vi "bead-center-xy-correlation-simple-sum-v3.vi"(4 "Radial size":i32=64, 6 "Bead\nCoordinates":i32[](array[numeric])=[257, 440, 328, 479], 8 "error in (no error)":errorcluster caption="错误输入（无错误）", 9 "Scan Window Size":i32=40, 10 "Lines amount":i32=20, 11 "FullImage":T1) -> (0 "error out":errorcluster caption="错误输出", 1 "CoordinatesOut":i32[](array[numeric]), 2 "xy":dbl[](array[numeric]))   [LabVIEW 2013]
uses:
  <vilib>/vision/Image Controls.llb/IMAQ Image.ctl
panel:
  in  "传递变量":T2={"FullImage"=refnum, "Lines amount"=20, "Scan Window Size"=40, "Bead\nCoordinates"=[257, 440, 328, 479], "Radial size"=64, "center_X"=0.0, "center_Y"=0.0, "再次确认ROI"=FALSE}
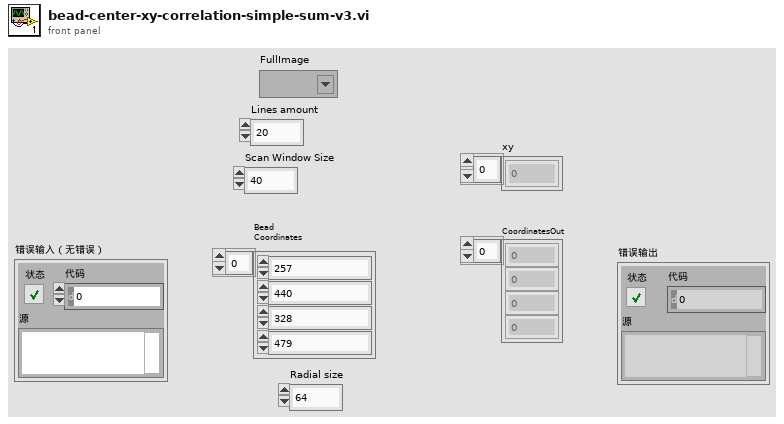
[diagram p1: front panel]
types:
  T1 = typedef "IMAQ Image.ctl" = refnum<image>
  T2 = cluster{"FullImage":T1, "Lines amount":i32, "Scan Window Size":i32, "Bead\nCoordinates":i32[], "Radial size":i32, "center_X":dbl, "center_Y":dbl, "再次确认ROI":bool}
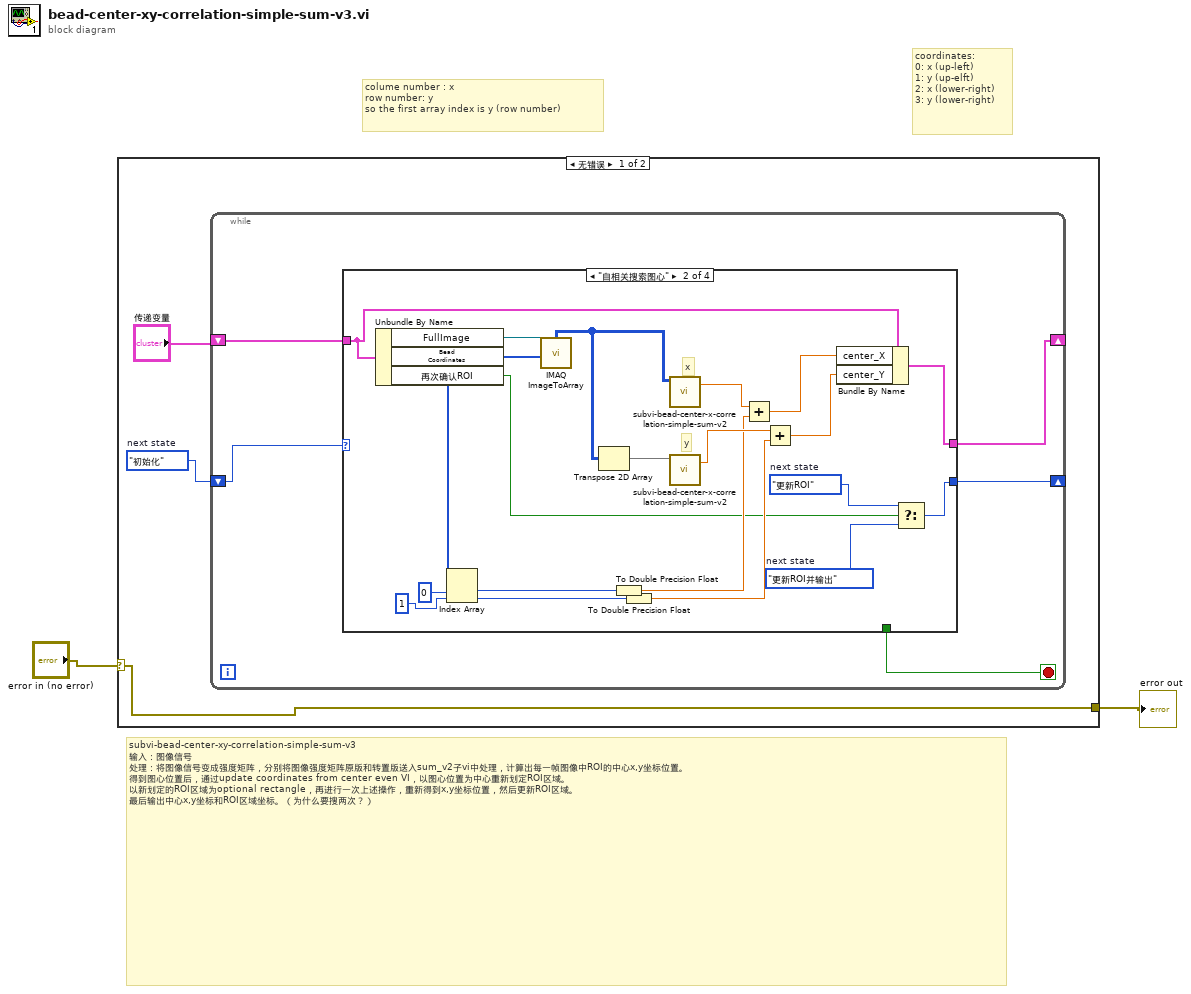
[diagram p0: block diagram]
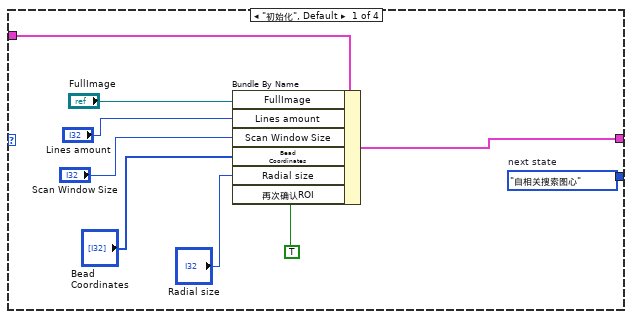
[diagram p2: hidden frame]
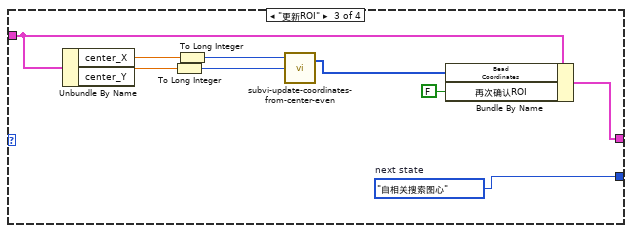
[diagram p3: hidden frame]
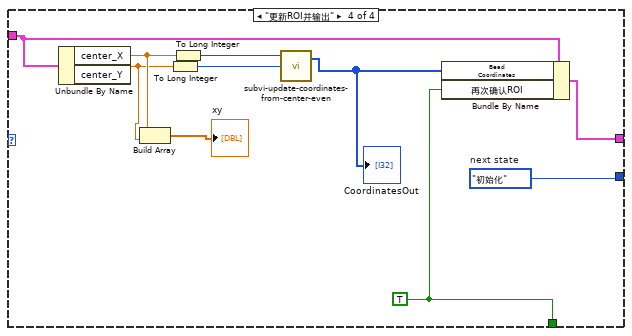
[diagram p4: hidden frame]
diagram:
  # "colume number : x\nrow number: y\nso the first array index is y (row number)"
  # "coordinates:\n0: x (up-left)\n1: y (up-elft)\n2: x (lower-right)\n3: y (lower-right)"
  # "subvi-bead-center-xy-correlation-simple-sum-v3\n输入：图像信号\n处理：将图像信号变成强度矩阵，分别将图像强度矩阵原版和转置版送入sum_v2子vi中处理，计算出每一帧图像中ROI的中心x,y坐标位置。\n得到图心位置后，通过update coordinates from center even VI，以图心位置为中心重新划定ROI区域。\n以新划定的ROI区域为optional rectangle，再进行一次上述操作，重新得到x,y坐标位置，然后更新ROI区域。\n最后输出中心x,y坐标和ROI区域坐标。（为什么要搜两次？）"
  n1 = case shown="无错误" "error in (no error)" {
    selector: "error in (no error)" -> [w5 w59]
    tunnel: [w5 w59] -> w1
    frame No Error {
      w3 = enum16{"初始化", "自相关搜索图心", "更新ROI", "更新ROI并输出"}."初始化"  # next state
      n2 = while {
        shift-right: [w9] -> _
        shift-left: "传递变量" -> [w10]
        shift-right: [w7] -> _
        shift-left: w3 -> [w8]
        stop <- w6 stop-if-true
        n3 = case shown="\"自相关搜索图心\"" w8 {
          tunnel: w10 -> [w19 w30 w44 w56]
          tunnel: [w13 w25 w42 w54] -> w9
          tunnel: [w12 w23 w41 w55] -> w7
          tunnel: [_ _ _ w49] -> w6
          frame "初始化", Default {
            w12 = enum16{"初始化", "自相关搜索图心", "更新ROI", "更新ROI并输出"}."自相关搜索图心"  # next state
            n4 = Bundle By Name(cluster=w19, "FullImage"="FullImage", "Lines amount"="Lines amount", "Scan Window Size"="Scan Window Size", "Bead\nCoordinates"="Bead\nCoordinates", "Radial size"="Radial size", "再次确认ROI"=TRUE) -> (w13:T2)
          }
          frame "自相关搜索图心" {
            w22 = enum16{"初始化", "自相关搜索图心", "更新ROI", "更新ROI并输出"}."更新ROI并输出"  # next state
            w24 = enum16{"初始化", "自相关搜索图心", "更新ROI", "更新ROI并输出"}."更新ROI"  # next state
            # "y"
            # "x"
            n5 = Unbundle By Name(w30) -> ("FullImage"=w33:T1, "Bead\nCoordinates"=w20:i32[], "再次确认ROI"=w21:bool)
            n6 = Index Array(array=w20, index #1=0 ("index"), index #2=1 ("index")) -> (element #1=w32:i32, element #2=w31:i32)
            n7 = call "IMAQ ImageToArray"("Optional Rectangle"=w20, "Image"=w33) -> ("Image Pixels (U8)"=w39:u8[][])  [unwired: 1 in, 5 out]
            n8 = Transpose 2D Array(2D array=w39) -> (transposed array=w38:u8[][])
            n9 = To Double Precision Float(number=w32) -> (double precision float=w27:dbl)
            n10 = To Double Precision Float(number=w31) -> (double precision float=w26:dbl)
            n11 = call "subvi-bead-center-x-correlation-simple-sum-v2.vi"("Image Pixels (U8)"=w39) -> ("center coordinate x"=w37:dbl)  [unwired: 3 in, 1 out]
            n12 = call "subvi-bead-center-x-correlation-simple-sum-v2.vi"("Image Pixels (U8)"=w38) -> ("center coordinate x"=w36:dbl)  [unwired: 3 in, 1 out]
            n13 = Add(x=w37, y=w27) -> (x+y=w29:dbl)
            n14 = Add(x=w36, y=w26) -> (x+y=w28:dbl)
            n15 = Bundle By Name(cluster=w30, "center_X"=w29, "center_Y"=w28) -> (w25:T2)
            n16 = Select(t=w24, s=w21, f=w22) -> (s? t:f=w23:enum16{"初始化", "自相关搜索图心", "更新ROI", "更新ROI并输出"})
          }
          frame "更新ROI" {
            w41 = enum16{"初始化", "自相关搜索图心", "更新ROI", "更新ROI并输出"}."自相关搜索图心"  # next state
            n17 = Unbundle By Name(w44) -> ("center_X"=w48:dbl, "center_Y"=w47:dbl)
            n18 = To Long Integer(number=w47) -> (32bit integer=w45:i32)
            n19 = To Long Integer(number=w48) -> (32bit integer=w46:i32)
            n20 = call "subvi-update-coordinates-from-center-even.vi"("center_y"=w45, "center_x"=w46) -> ("CoordinatesOut"=w43:i32[])  [unwired: 1 in, 1 out]
            n21 = Bundle By Name(cluster=w44, "Bead\nCoordinates"=w43, "再次确认ROI"=FALSE) -> (w42:T2)
          }
          frame "更新ROI并输出" {
            w49 = TRUE
            w55 = enum16{"初始化", "自相关搜索图心", "更新ROI", "更新ROI并输出"}."初始化"  # next state
            n22 = Unbundle By Name(w56) -> ("center_X"=w51:dbl, "center_Y"=w50:dbl)
            n23 = Build Array(w51, w50) -> (→"xy":dbl[])
            n24 = To Long Integer(number=w50) -> (32bit integer=w58:i32)
            n25 = To Long Integer(number=w51) -> (32bit integer=w57:i32)
            n26 = call "subvi-update-coordinates-from-center-even.vi"("center_y"=w58, "center_x"=w57) -> ("CoordinatesOut"=w53:i32[])  [unwired: 1 in, 1 out]
            "CoordinatesOut" <- w53
            n27 = Bundle By Name(cluster=w56, "Bead\nCoordinates"=w53, "再次确认ROI"=w49) -> (w54:T2)
          }
        }
      }
    }
    frame Error {
    }
  }
  "error out" <- w1
